vi "SMTP Email Transliterate Settings.vi"(4 "transliteration":string, 5 "character set":string) -> (0 "map":u8[](array[numeric]), 1 "charset out":string)   [LabVIEW 2011, in "NewNI_SMTPEmail.lvlib"]
doc: "Maintains the default settings for the SMTP VIs. When function is \"use\", any of the return address, subject, server, and character set inputs that are not empty are left unaffected, the ones that are empty are replaced by default settings.\n\nfunction - specifies action to perform (default use)\n use - rpelaces empty inputs with defaults and returns them in return address out, subject out, server out, and chatacter set out. Also returns a mapping to be applied for text messages.\n set - sets the default settings to be return address, subject, server, and character set. Also loads transliteration tables based on transliteration.\n read ini - sets the default settings from the SMTP.ini file\n\nreturn address - return address to be used (default from SMTP.ini)\n\nsubject - subject to be used (default from SMTP.ini)\n\nserver - SMTP server to be used (default from SMTP.ini)\n\ncharacter set - return address to be used (default from SMTP.ini)\n\ntransliteration - (with set) specifies which transliteration tables to load\n\nmap - (with use) specifies how characters should be mapped"
uses:
  NewNI_SMTPEmail.lvlib
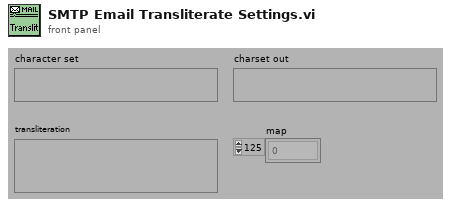
[diagram p1: front panel]
types:
  T1 = typedef "NewNI_SMTPEmail.lvlib/SMTP Email Keyed Array.ctl" = cluster{"keys":string[], "values":string[]}
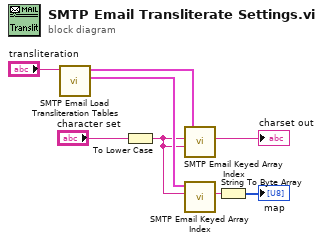
[diagram p0: block diagram]
diagram:
  n1 = call "SMTP Email Load Transliteration Tables.vi"("\"Transliterate\" config"="transliteration") -> ("maps"=w6:T1, "charsets"=w7:T1)  [unwired: 5 out]
  n2 = To Lower Case(string="character set") -> (all lower case string=w2:string)
  n3 = call "SMTP Email Keyed Array Index.vi"("default value"=w2, "key"=w2, "array in"=w7) -> ("value"=→"charset out":string)  [unwired: 1 in, 3 out]
  n4 = call "SMTP Email Keyed Array Index.vi"("key"=w2, "array in"=w6) -> ("value"=w5:string)  [unwired: 2 in, 3 out]
  n5 = String To Byte Array(string=w5) -> (unsigned byte array=→"map":u8[])
